vi "Launch Async Calculator.vi"(8 "error in (no error)":errorcluster, 10 "Calculation Period (ms)":u32, 11 "Load Calculator in":refnum<class "CANBus_Load_Calculator.lvclass">) -> (0 "error out":errorcluster, 3 "Load Calculator out":refnum<class "CANBus_Load_Calculator.lvclass">)   [LabVIEW 2018, in "NI-XNET Monitor Engine.lvlib" / "XNET-Bus-Load-Calculator.lvlib" / "CANBus_Load_Calculator.lvclass"]
uses:
  CANBus_Load_Calculator.lvclass
  CANBus_Load_Calculator.lvclass/CANBus_Load_Calculator.ctl
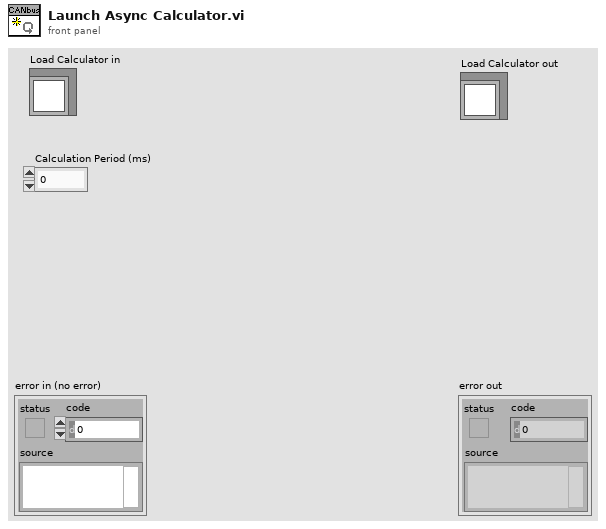
[diagram p1: front panel]
types:
  T1 = typedef "NI-XNET Monitor Engine.lvlib/XNET-Bus-Load-Calculator.lvlib/CANBus_Load_Calculator.lvclass/Calc_Comm_Refs.ctl" = cluster{"ToCalculator_QRef":refnum<queue>, "FromCalculator_QRef":refnum<queue>}
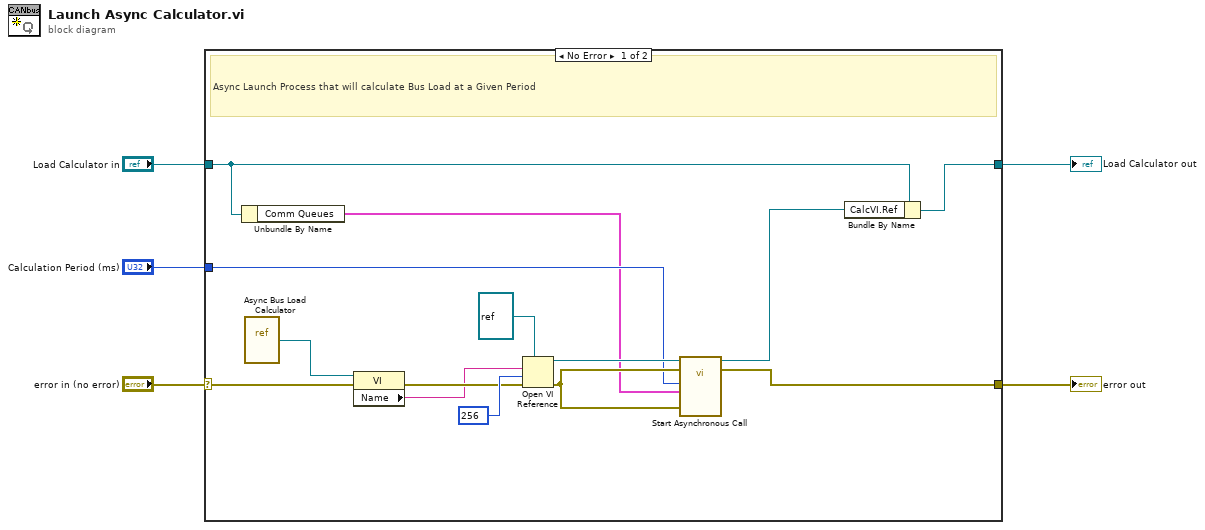
[diagram p0: block diagram]
diagram:
  n1 = case shown="No Error" "error in (no error)" {
    selector: "error in (no error)" -> [w12 w21]
    tunnel: [w10 w21] -> w4
    tunnel: "Load Calculator in" -> [w9 w20]
    tunnel: [w8 w20] -> w2
    tunnel: "Calculation Period (ms)" -> [w11 _]
    frame No Error {
      # "Async Launch Process that will calculate Bus Load at a Given Period"
      n2 = Unbundle By Name(w9) -> ("Comm Queues"=w7:T1)
      n3 = vi-ref "Async Bus Load Calculator.vi"() -> (w18:refnum<vi>)
      n4 = property class="VI"(reference=w18, error in=w12) -> (error out=w17:errorcluster, "Name"=w16:string)  [unwired: 1 out]
      n5 = Open VI Reference(type specifier VI Refnum (for type only)=refnum<vi> refnum, vi path=w16, options=256, error in (no error)=w17) -> (vi reference=w14:refnum<vi>, error out=w13:errorcluster)  [unwired: 2 in]
      n6 = call-by-ref "Start Asynchronous Call"(reference=w14, error in=w13, 8:"error in (no error)"=w13, "Comm Queues"=w7, "Calculation Period (ms)"=w11) -> (reference out=w6:refnum<vi>, error out=w10:errorcluster)  [unwired: 8 in, 1 out]
      n7 = Bundle By Name(cluster=w9, "CalcVI.Ref"=w6) -> (w8:refnum<class "CANBus_Load_Calculator.lvclass">)
    }
    frame Error {
    }
  }
  "error out" <- w4
  "Load Calculator out" <- w2
